vi "Process Data Conifg PID 0 Data line_vel.vi"(11 "출력 클러스터 2":T2) -> (2 "Pos PID gain 0":T1, 3 "Velocity limit 0":cluster{"output high":dbl, "output low":dbl})   [LabVIEW 2019]
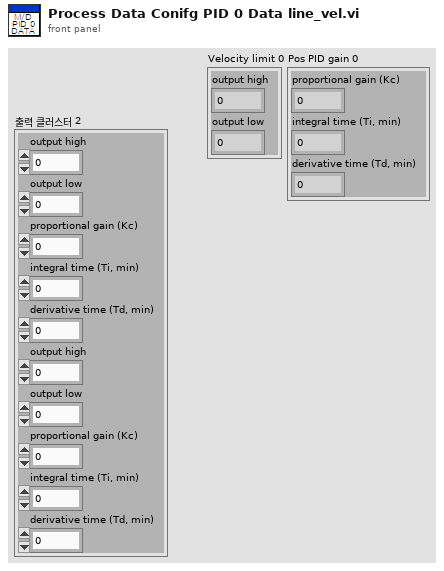
[diagram p1: front panel]
types:
  T1 = cluster{"proportional gain (Kc)":dbl, "integral time (Ti, min)":dbl, "derivative time (Td, min)":dbl}
  T2 = cluster{"output high":dbl, "output low":dbl, "proportional gain (Kc)":dbl, "integral time (Ti, min)":dbl, "derivative time (Td, min)":dbl, "output high":dbl, "output low":dbl, "proportional gain (Kc)":dbl, "integral time (Ti, min)":dbl, "derivative time (Td, min)":dbl}
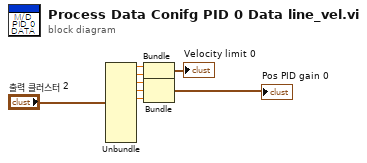
[diagram p0: block diagram]
diagram:
  n1 = Unbundle("출력 클러스터 2") -> ("output high"=w5:dbl, "output low"=w4:dbl, "proportional gain (Kc)"=w6:dbl, "integral time (Ti, min)"=w7:dbl, "derivative time (Td, min)"=w8:dbl)  [unwired: 5 out]
  n2 = Bundle("output high"=w5, "output low"=w4) -> (→"Velocity limit 0":cluster{"output high":dbl, "output low":dbl})  [unwired: 1 in]
  n3 = Bundle("proportional gain (Kc)"=w6, "integral time (Ti, min)"=w7, "derivative time (Td, min)"=w8) -> (→"Pos PID gain 0":T1)  [unwired: 1 in]
